vi "widthCalculate.vi"(4 "time_B_noInter":dbl[](array[numeric]), 5 "Error In":errorcluster, 6 "VE_B_noInter":dbl[](array[numeric]), 7 "time_B":dbl[](array[numeric]), 8 "VE_B":dbl[](array[numeric])) -> (0 "Error Out":errorcluster, 1 "maxWidth":dbl format="%#.2g", 2 "noMin":bool, 3 "Ampl. (L/min)":dbl format="%#.2g")   [LabVIEW 2012]
uses:
  <vilib>/measure/mamon.llb/Waveform Peak Detection for 1 Chan.vi
  <vilib>/Analysis/baseanly.llb/Mean (DBL).vi
  <vilib>/measure/NI_MAPro.lvlib
  <vilib>/Analysis/NI_AALBase.lvlib
panel:
  out "Ventilation":cluster{"Array":dbl[], "time_B":dbl[]}(graph)
  out "Duration (s)":dbl[](array[numeric]) format="%#.2g"
  out "Amplitude (L/min)":dbl[](array[numeric]) format="%#.2g"
  out "Freq. (1/min)":dbl format="%#.2g"
  out "EOB Ratio":dbl format="%#.2g"
  out "Cycles number:":i32
  out "iValesLocation":dbl[](array[numeric])
  out "valesAmplitude":dbl[](array[numeric])
  out "peaksAmplitude":dbl[](array[numeric])
  out "iPeaksLocation":dbl[](array[numeric])
  in  "Threshold (L/min):":dbl=1.0
  out "filteredSignal":dbl[](array[numeric])
  out "lastTime":dbl format="%#.6g"
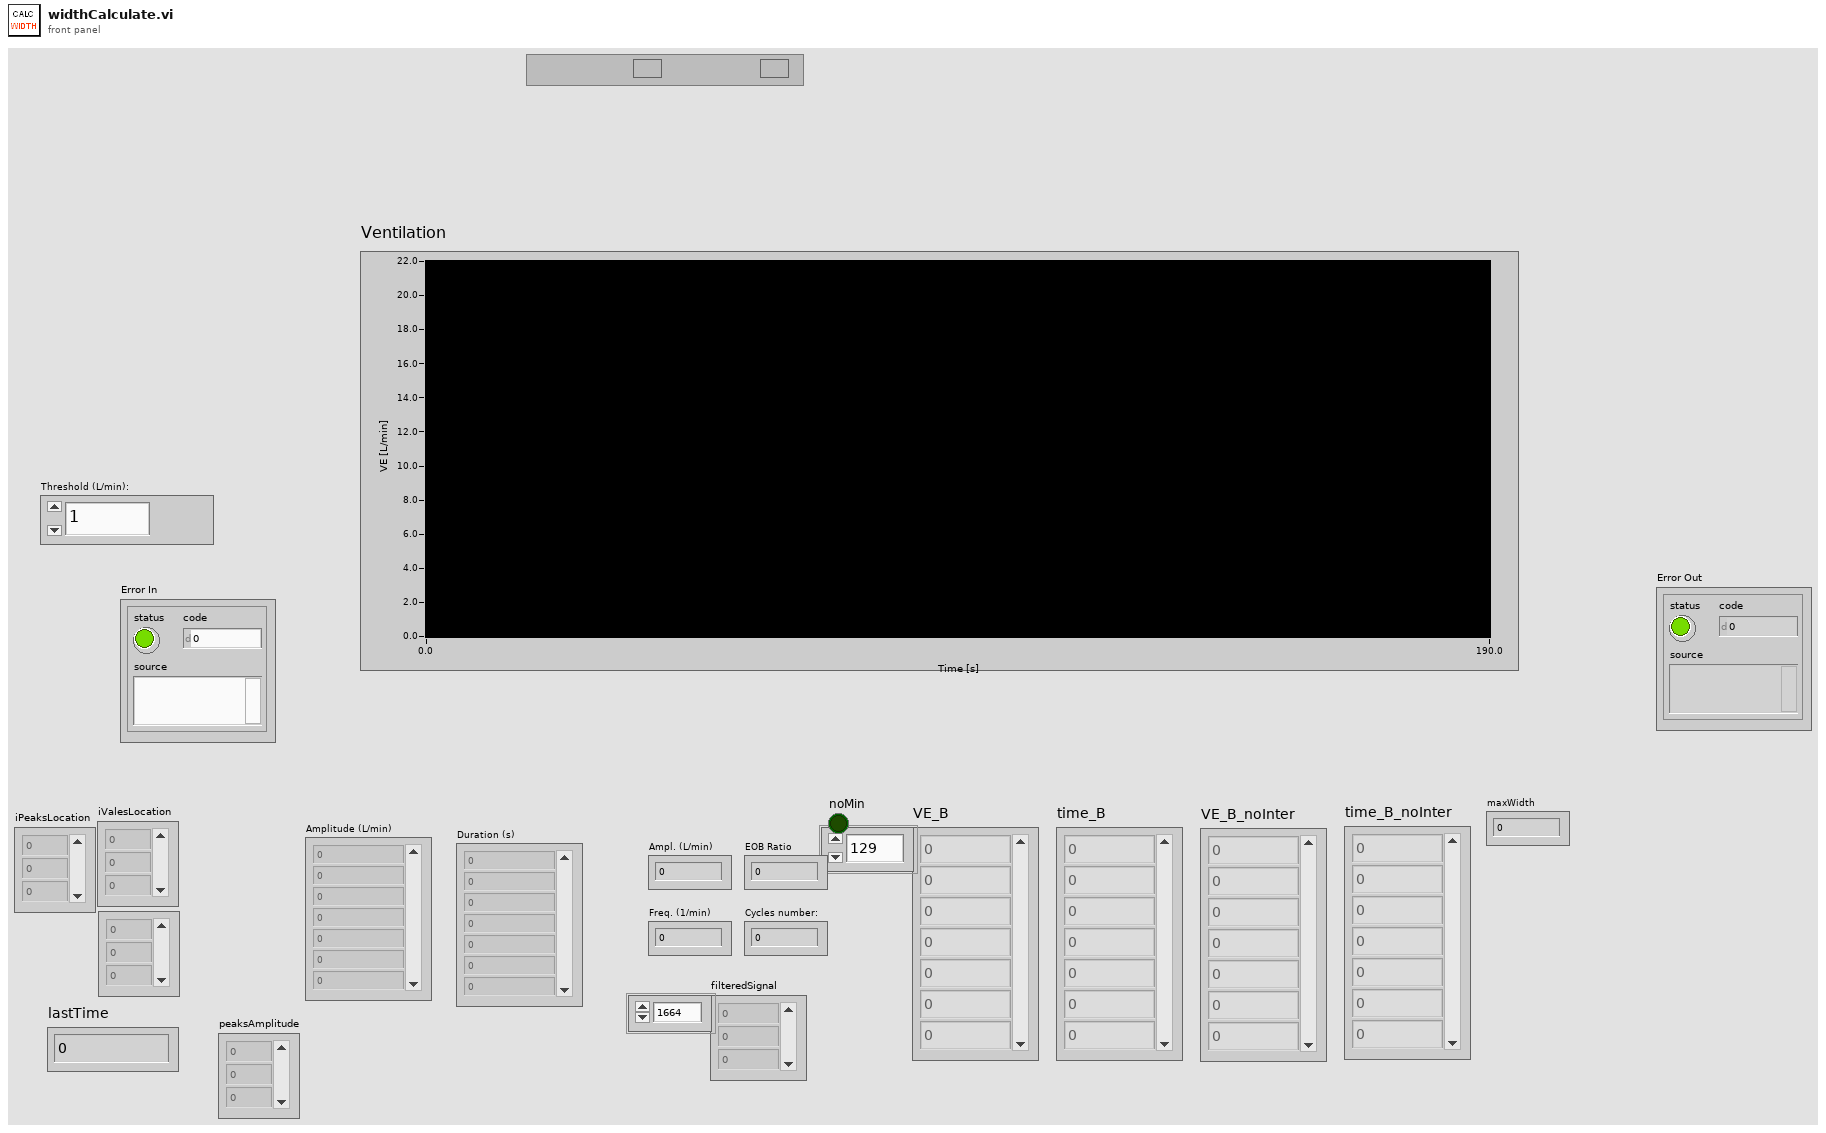
[diagram p1: front panel]
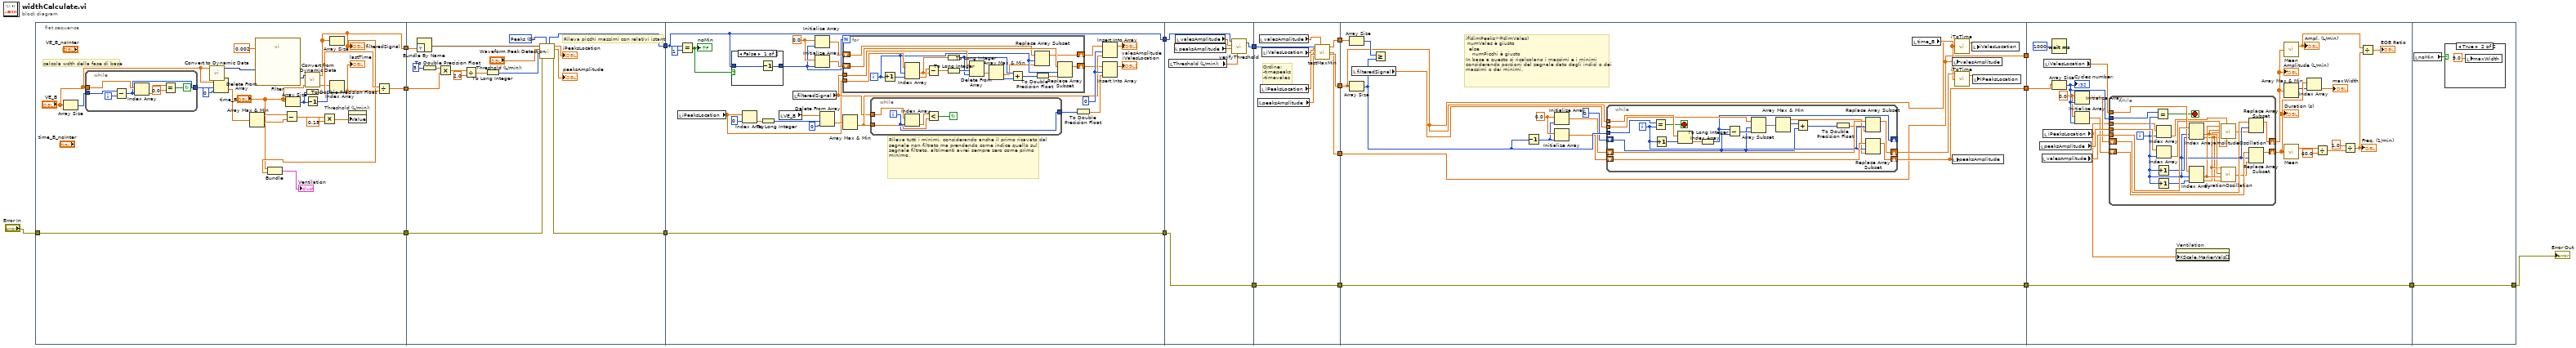
[diagram p0: block diagram]
diagram:
  n1 = flat-sequence {
    tunnel: [w41] -> w19
    tunnel: [w22] -> w18
    tunnel: [w20] -> w9
    tunnel: "Error In" -> [w20]
    tunnel: [w64] -> w17
    tunnel: w19 -> [w58]
    tunnel: w18 -> [w63]
    tunnel: w9 -> [w50]
    tunnel: [w49] -> w7
    tunnel: w17 -> [w66]
    tunnel: [w66] -> w16
    tunnel: w7 -> [w65]
    tunnel: [w65] -> w6
    tunnel: w16 -> [w120]
    tunnel: [w117] -> w15
    tunnel: w6 -> [w116]
    tunnel: [w116] -> w3
    tunnel: w15 -> [w129]
    tunnel: [w126] -> w14
    tunnel: [w125] -> w13
    tunnel: [w122] -> w12
    tunnel: [w121] -> w4
    tunnel: w3 -> [w121]
    tunnel: w14 -> [w136]
    tunnel: w13 -> [w137]
    tunnel: [w139] -> w11
    tunnel: [w138] -> w10
    tunnel: w12 -> [w138]
    tunnel: [w130] -> w5
    tunnel: w4 -> [w130]
    tunnel: w10 -> [_]
    tunnel: w11 -> [w168]
    tunnel: w5 -> [w166]
    tunnel: [w166] -> w2
    tunnel: w2 -> [w209]
    tunnel: [w209] -> w1
    frame #0 {
      # "calcola wdth della fase di base"
      n2 = Array Size(array="VE_B") -> (size(s)=w28:i32)
      n3 = while {
        tunnel: "VE_B" -> [w48]
        tunnel: w28 -> [w47]
        tunnel: [w42] -> w27
        i -> [w46]
        stop <- w43 continue-if-true
        n4 = Subtract(x=w47, y=w46) -> (x-y=w42:i32)
        n5 = Index Array(array=w48, index=w42) -> (element=w45:dbl)
        n6 = Equal?(x=w45, y=0.0) -> (x = y?=w43:bool)
      }
      n7 = call "Convert to Dynamic Data"("Array"="VE_B") -> ("Dynamic Data Type"=w40:dynamicdata)  [unwired: 3 in]
      n8 = Delete From Array(array="VE_B", length=w27, index=0) -> (deleted portion=w25:dbl[])  [unwired: 1 out]
      n9 = Array Max & Min(array=w25) -> (max value=w33:dbl, min value=w32:dbl)  [unwired: 2 out]
      n10 = call "Filter"("Lower Cut-Off"=0.002 ("Low Cut-off (Hz):"), "Signal"=w40) -> ("Filtered Signal"=w39:dynamicdata)  [unwired: 8 in, 1 out]
      n11 = Subtract(x=w33, y=w32) -> (x-y=w31:dbl)
      n12 = Array Size(array="time_B") -> (size(s)=w35:i32)
      n13 = call "Convert from Dynamic Data"("Dynamic Data Type"=w39) -> ("Array"=w22:dbl[])  [unwired: 3 in]
      "filteredSignal" <- w22
      n14 = Bundle("time_B"="time_B", "Array"=w22) -> (→"Ventilation":cluster{"time_B":dbl[], "Array":dbl[]})  [unwired: 1 in]
      n15 = To Double Precision Float(number=w35) -> (double precision float=w36:dbl)
      n16 = Decrement(x=w35) -> (x-1=w37:i32)
      n17 = Multiply(x=w31, y=0.15) -> (x*y=w29:dbl)
      n18 = Array Size(array=w22) -> ()  [unwired: 1 out]
      n19 = Index Array(array="time_B", index=w37) -> (element=w34:dbl)
      "lastTime" <- w34
      n20 = property on="Threshold (L/min):" class="DigNum (strict)"("Value"=w29) -> ()  [unwired: 2 in, 2 out]
      n21 = Divide(x=w36, y=w34) -> (x/y=w41:dbl)
    }
    frame #1 {
      w61 = u16 0 items=["Peaks", "Valleys"] ("peaks/valleys")
      # "Rileva picchi massimi con relativi istanti"
      n22 = Bundle By Name("Y"=w63) -> (w60:waveform(dbl))  [unwired: 1 in]
      n23 = To Double Precision Float(number=5 ("Width (s):")) -> (double precision float=w57:dbl)
      n24 = Multiply(x=w57, y=w58) -> (x*y=w56:dbl)
      n25 = Divide(x=w56, y=2.0) -> (x/y=w54:dbl)
      n26 = To Long Integer(number=w54) -> (32bit integer=w52:i32)
      n27 = call-poly <vilib>:"Waveform Peak Detection.vi"("peaks/valleys"=w61, "error in"=w50, "width"=w52, "threshold"="Threshold (L/min):", "Signal In"=w60) -> ("error out"=w49:errorcluster, "Amplitudes"=→"peaksAmplitude":dbl[], "Locations"=→"iPeaksLocation":dbl[], "# found"=w64:i32)  [unwired: 2 in, 1 out]
    }
    frame #2 {
      w81 = 0 ("index")
      w83 = 0.0 ("element")
      # "Rileva tutti i minimi, considerando anche il primo ricavato dal segnale non filtrato ma prendendo come indice quello sul \nsegnale filtrato, altrimenti avrei sempre zero come primo minimo."
      n28 = local read "iPeaksLocation"() -> (w73:dbl[])
      n29 = Equal?(x=w66, y=1) -> (x = y?=w69:bool)
      "noMin" <- w69
      n30 = case shown="False" w69 {
        tunnel: w66 -> [w90 w91]
        tunnel: [w89 w91] -> w67
        frame False {
          n31 = Decrement(x=w90) -> (x-1=w89:i32)
        }
        frame True {
        }
      }
      n32 = Index Array(array=w73, index=0) -> (element=w86:dbl)
      n33 = To Long Integer(number=w86) -> (32bit integer=w78:i32)
      n34 = local read "VE_B"() -> (w88:dbl[])
      n35 = local read "filteredSignal"() -> (w74:dbl[])
      n36 = Initialize Array(w83, w67) -> (w68:dbl[])
      n37 = Initialize Array(w83, w67) -> (w75:dbl[])
      n38 = Delete From Array(array=w88, length=w78, index=0) -> (deleted portion=w84:dbl[])  [unwired: 1 out]
      n39 = for {
        N: w67 -> [_]
        tunnel: w74 -> [w109]
        tunnel: w73 -> [w108]
        shift-right: [w100] -> w71
        shift-left: w75 -> [w101]
        shift-right: [w98] -> w72
        shift-left: w68 -> [w99]
        i -> [w94]
        n40 = Increment(x=w94) -> (x+1=w107:i32)
        n41 = Index Array(array=w108, index #1=w94, index #2=w107) -> (element #1=w105:dbl, element #2=w106:dbl)
        n42 = Subtract(x=w106, y=w105) -> (x-y=w104:dbl)
        n43 = To Long Integer(number=w105) -> (32bit integer=w95:i32)
        n44 = To Long Integer(number=w104) -> (32bit integer=w103:i32)
        n45 = Delete From Array(array=w109, length=w103, index=w95) -> (deleted portion=w102:dbl[])  [unwired: 1 out]
        n46 = Array Max & Min(array=w102) -> (min value=w93:dbl, min index (indices)=w97:i32)  [unwired: 2 out]
        n47 = Add(x=w95, y=w97) -> (x+y=w96:i32)
        n48 = Replace Array Subset(array=w99, new element=w93, index=w94) -> (w98:dbl[])
        n49 = To Double Precision Float(number=w96) -> (double precision float=w92:dbl)
        n50 = Replace Array Subset(array=w101, new element=w92, index=w94) -> (w100:dbl[])
      }
      n51 = Array Max & Min(array=w84) -> (min value=w79:dbl)  [unwired: 3 out]
      n52 = while {
        tunnel: w79 -> [w112]
        tunnel: w74 -> [w114]
        tunnel: [w110] -> w77
        i -> [w110]
        stop <- w111 continue-if-true
        n53 = Index Array(array=w114, index=w110) -> (element=w113:dbl)
        n54 = Less?(x=w113, y=w112) -> (x < y?=w111:bool)
      }
      n55 = To Double Precision Float(number=w77) -> (double precision float=w76:dbl)
      n56 = Insert Into Array(array=w72, index=w81, new element=w79) -> (→"valesAmplitude":dbl[])
      n57 = Insert Into Array(array=w71, index=w81, new element=w76) -> (→"iValesLocation":dbl[])
    }
    frame #3 {
      n58 = local read "Threshold (L/min):"() -> (w115:dbl)
      n59 = local read "peaksAmplitude"() -> (w118:dbl[])
      n60 = local read "valesAmplitude"() -> (w119:dbl[])
      n61 = call "verifyThreshold.vi"("#Peaks"=w120, "valesAmplitude"=w119, "peaksAmplitude"=w118, "threshold"=w115) -> ("passThreshold"=w117:i32[])  [unwired: 1 in, 1 out]
    }
    frame #4 {
      # "Ordine:\n-timepeaks\n-timevales"
      n62 = local read "peaksAmplitude"() -> (w123:dbl[])
      n63 = local read "valesAmplitude"() -> (w124:dbl[])
      n64 = local read "iPeaksLocation"() -> (w127:dbl[])
      n65 = local read "iValesLocation"() -> (w128:dbl[])
      n66 = call "testMaxMin.vi"("valesAmplitude in"=w124, "peaksAmplitude in"=w123, "iPeaksLocation in"=w127, "iValesLocation in"=w128, "passThreshold"=w129) -> ("iValesLocation out"=w125:dbl[], "iPeaksLocation out"=w126:dbl[], "valesAmplitude out"=w122:dbl[])  [unwired: 1 in, 2 out]
    }
    frame #5 {
      w133 = 0.0 ("element")
      # "if(dimPeaks>=dimVales)\n numVales è giusto\n  else\n    numPicchi è giusto\nIn base a questo si ricalcolano i massimi e i minimi considerando porzioni del segnale dato dagli indici o dei massimi o dei minimi."
      n67 = Array Size(array=w136) -> (size(s)=w143:i32)
      n68 = Array Size(array=w137) -> (size(s)=w146:i32)
      n69 = local read "filteredSignal"() -> (w145:dbl[])
      n70 = Greater Or Equal?(x=w143, y=w146) -> ()  [unwired: 1 out]
      n71 = Decrement(x=w146) -> (x-1=w132:i32)
      n72 = Initialize Array(w133, w132) -> (w131:dbl[])
      n73 = Initialize Array(w133, w132) -> (w134:dbl[])
      n74 = while {
        tunnel: w137 -> [w165]
        tunnel: w146 -> [w164]
        tunnel: w145 -> [w161]
        shift-right: [w147] -> _
        shift-left: 0 -> [w148]
        shift-right: [w158] -> w139
        shift-left: w134 -> [w159]
        shift-right: [w156] -> w144
        shift-left: w131 -> [w157]
        i -> [w155]
        stop <- w163 stop-if-true
        n75 = Equal?(x=w164, y=w155) -> (x = y?=w163:bool)
        n76 = Increment(x=w155) -> (x+1=w151:i32)
        n77 = Index Array(array=w165, index=w151) -> (element=w162:dbl)
        n78 = To Long Integer(number=w162) -> (32bit integer=w147:i32)
        n79 = Subtract(x=w147, y=w148) -> (x-y=w149:i32)
        n80 = Array Subset(array=w161, index=w148, length=w149) -> (w160:dbl[])
        n81 = Array Max & Min(array=w160) -> (max value=w153:dbl, max index (indices)=w154:i32)  [unwired: 2 out]
        n82 = Add(x=w154, y=w148) -> (x+y=w150:i32)
        n83 = To Double Precision Float(number=w150) -> (double precision float=w152:dbl)
        n84 = Replace Array Subset(array=w157, new element=w152, index=w155) -> (w156:dbl[])
        n85 = Replace Array Subset(array=w159, new element=w153, index=w155) -> (w158:dbl[])
      }
      n86 = local read "time_B"() -> (w141:dbl[])
      n87 = local write "peaksAmplitude"(w139) -> ()
      n88 = local write "valesAmplitude"(w138) -> ()
      n89 = call "iToTime.vi"("time"=w141, "iArray"=w137) -> ("timeArray"=w142:dbl[])  [unwired: 1 in, 1 out]
      n90 = call "iToTime.vi"("time"=w141, "iArray"=w144) -> ("timeArray"=w140:dbl[])  [unwired: 1 in, 1 out]
      n91 = local write "iValesLocation"(w142) -> ()
      n92 = local write "iPeaksLocation"(w140) -> ()
    }
    frame #6 {
      w184 = 0.0 ("element")
      n93 = local read "peaksAmplitude"() -> (w187:dbl[])
      n94 = local read "valesAmplitude"() -> (w186:dbl[])
      n95 = local read "iPeaksLocation"() -> (w167:dbl[])
      n96 = local read "iValesLocation"() -> (w180:dbl[])
      n97 = Wait (ms)(milliseconds to wait=u32 1000) -> ()  [unwired: 1 out]
      n98 = Array Size(array=w168) -> (size(s)=w185:i32)
      "Cycles number:" <- w185
      n99 = Initialize Array(w184, w185) -> (w183:dbl[])
      n100 = Initialize Array(w184, w185) -> (w182:dbl[])
      n101 = while {
        tunnel: w187 -> [w208]
        tunnel: w167 -> [w188]
        tunnel: w186 -> [w207]
        tunnel: w180 -> [w206]
        tunnel: w185 -> [w205]
        shift-right: [w198] -> w171
        shift-left: w182 -> [w199]
        shift-right: [w200] -> w172
        shift-left: w183 -> [w201]
        i -> [w197]
        stop <- w204 stop-if-true
        n102 = Equal?(x=w205, y=w197) -> (x = y?=w204:bool)
        n103 = Increment(x=w197) -> (x+1=w203:i32)
        n104 = Increment(x=w197) -> (x+1=w202:i32)
        n105 = Index Array(array=w188, index=w197) -> (element=w195:dbl)
        n106 = Index Array(array=w208, index=w197) -> (element=w194:dbl)
        n107 = Index Array(array=w207, index #1=w197, index #2=w203) -> (element #1=w192:dbl, element #2=w190:dbl)
        n108 = Index Array(array=w206, index #1=w197, index #2=w202) -> (element #1=w193:dbl, element #2=w191:dbl)
        n109 = call "amplitudeOscillation.vi"("y0"=w194, "x0"=w195, "y2"=w190, "x2"=w191, "y1"=w192, "x1"=w193) -> ("amplitudeOscillation"=w189:dbl)
        n110 = call "durationOscillation.vi"("valesAmplitude2"=w190, "timeValesLocation1"=w193, "valesAmplitude1"=w192, "timeValesLocation2"=w191) -> ("durationOscilation"=w196:dbl)
        n111 = Replace Array Subset(array=w201, new element=w189, index=w197) -> (w200:dbl[])
        n112 = Replace Array Subset(array=w199, new element=w196, index=w197) -> (w198:dbl[])
      }
      "Duration (s)" <- w171
      "Amplitude (L/min)" <- w172
      n113 = property on="Ventilation" class="XYGraph (strict)"("XScale.MarkerVals[]"=w167) -> ()  [unwired: 2 in, 2 out]
      n114 = call-poly <vilib>:"Mean.vi"("X"=w172) -> ("mean"=w176:dbl)  [unwired: 1 out]
      "Ampl. (L/min)" <- w176
      n115 = Array Max & Min(array=w172) -> (max index (indices)=w170:i32)  [unwired: 3 out]
      n116 = call-poly <vilib>:"Mean.vi"("X"=w171) -> ("mean"=w173:dbl)  [unwired: 1 out]
      n117 = Index Array(array=w171, index=w170) -> (element=→"maxWidth":dbl)
      n118 = Divide(x=w173, y=60.0) -> (x/y=w178:dbl)
      n119 = Divide(x=1.0, y=w178) -> (x/y=w175:dbl)
      "Freq. (1/min)" <- w175
      n120 = Divide(x=w176, y=w175) -> (x/y=→"EOB Ratio":dbl)
    }
    frame #7 {
      n121 = local read "noMin"() -> (w210:bool)
      n122 = case shown="True" w210 {
        frame False {
        }
        frame True {
          n123 = local write "maxWidth"(9.0 ("maxWidth")) -> ()
        }
      }
    }
  }
  "Error Out" <- w1
